vi "Configure TrigLevel Core.vi"(8 "error in (no error)":errorcluster, 10 "TrigLvl":dbl[unit], 11 "CS++MCS in":refnum<class "CS++MCS.lvclass">) -> (0 "error out":errorcluster, 3 "CS++MCS out":refnum<class "CS++MCS.lvclass">)   [LabVIEW 2015, in "CS++MCS.lvlib" / "CS++MCS.lvclass"]
doc: "This VI configures the Trigger level used for analog triggering of the MCS."
uses:
  CS++MCS.lvclass
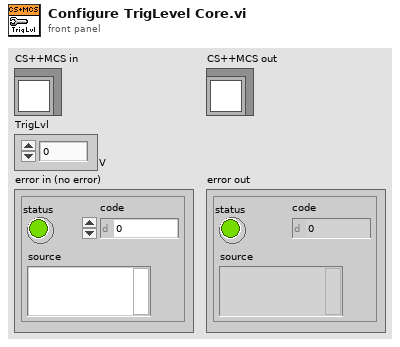
[diagram p1: front panel]
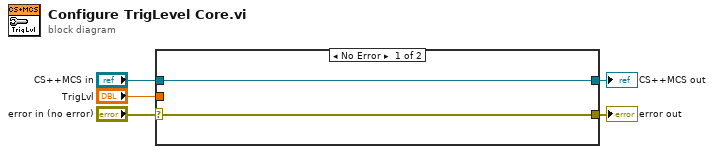
[diagram p0: block diagram]
diagram:
  n1 = case shown="No Error" "error in (no error)" {
    selector: "error in (no error)" -> [w6 w9]
    tunnel: [w6 w9] -> w4
    tunnel: [w7 w8] -> w2
    tunnel: "CS++MCS in" -> [w7 w8]
    tunnel: "TrigLvl" -> [_ _]
    frame No Error {
    }
    frame Error {
    }
  }
  "error out" <- w4
  "CS++MCS out" <- w2
